vi "svx_DAQ_ConvertState_1000toCurrent.vi"(10 "saved state (version 1.0.0.0)":T1, 11 "current state template":T2 caption="State" {"Timing Control 2" format="%#_6f"; "Channel Info Array"."Max" min=0.0 format="± %^#_4g"; "Channel Info Array"."Channel Type" items=["Voltage (V)"=0, "Charge (C)"=9, "-"=99, "SPL (Pa)"=3, "Force (lbf)"=6, "Force (N)"=1, "Acceleration (g) - IEPE"=2, "Acceleration (g) - Charge"=12, "Acceleration (g) - 4 wire DC Voltage"=22, "Velocity (in/s)"=7, "Velocity (mm/s)"=8, "Prox Probe (mil)"=4, "Prox Probe (mm)"=5]}) -> (3 "Default Control State out":T2 caption="State" {"Timing Control 2" format="%#_6f"; "Channel Info Array"."Max" min=0.0 format="± %^#_4g"; "Channel Info Array"."Channel Type" items=["Voltage (V)"=0, "Charge (C)"=9, "-"=99, "SPL (Pa)"=3, "Force (lbf)"=6, "Force (N)"=1, "Acceleration (g) - IEPE"=2, "Acceleration (g) - Charge"=12, "Acceleration (g) - 4 wire DC Voltage"=22, "Velocity (in/s)"=7, "Velocity (mm/s)"=8, "Prox Probe (mil)"=4, "Prox Probe (mm)"=5]})   [LabVIEW 2017, in "SVX NI-DAQmx AI Configuration XControl.xctl"]
uses:
  <vilib>/addons/Sound and Vibration/svt_DAQmx/Configuration XControl/SVX NI-DAQmx AI Configuration XControl.xctl
  <vilib>/addons/Sound and Vibration/svt_DAQmx/Configuration XControl/SubVIs/svx_DAQ_State.ctl
  <vilib>/addons/Sound and Vibration/svt_DAQmx/Configuration XControl/Controls/svx_DAQ_ChannelInfo.ctl
  <vilib>/addons/Sound and Vibration/svt_DAQmx/Configuration XControl/Controls/svx_DAQ_ChannelType.ctl
  <vilib>/addons/Sound and Vibration/svt_DAQmx/Configuration XControl/Controls/svx_DAQ_Coupling.ctl
  <vilib>/addons/Sound and Vibration/svt_DAQmx/Configuration XControl/Controls/svx_DAQ_Excitation.ctl
  <vilib>/addons/Sound and Vibration/svt_DAQmx/Configuration XControl/Controls/svx_DAQ_TimingType.ctl
  <vilib>/addons/Sound and Vibration/svt_DAQmx/Configuration XControl/Controls/svx_DAQ_ReferenceType.ctl
  <vilib>/addons/Sound and Vibration/svt_DAQmx/Configuration XControl/Controls/svx_DAQ_RotationDirection.ctl
  <vilib>/addons/Sound and Vibration/svt_DAQmx/Configuration XControl/Controls/svx_DAQ_Tach_Slope.ctl
  <vilib>/addons/Sound and Vibration/svt_DAQmx/Configuration XControl/Controls/svx_DAQ_Trigger_Slope.ctl
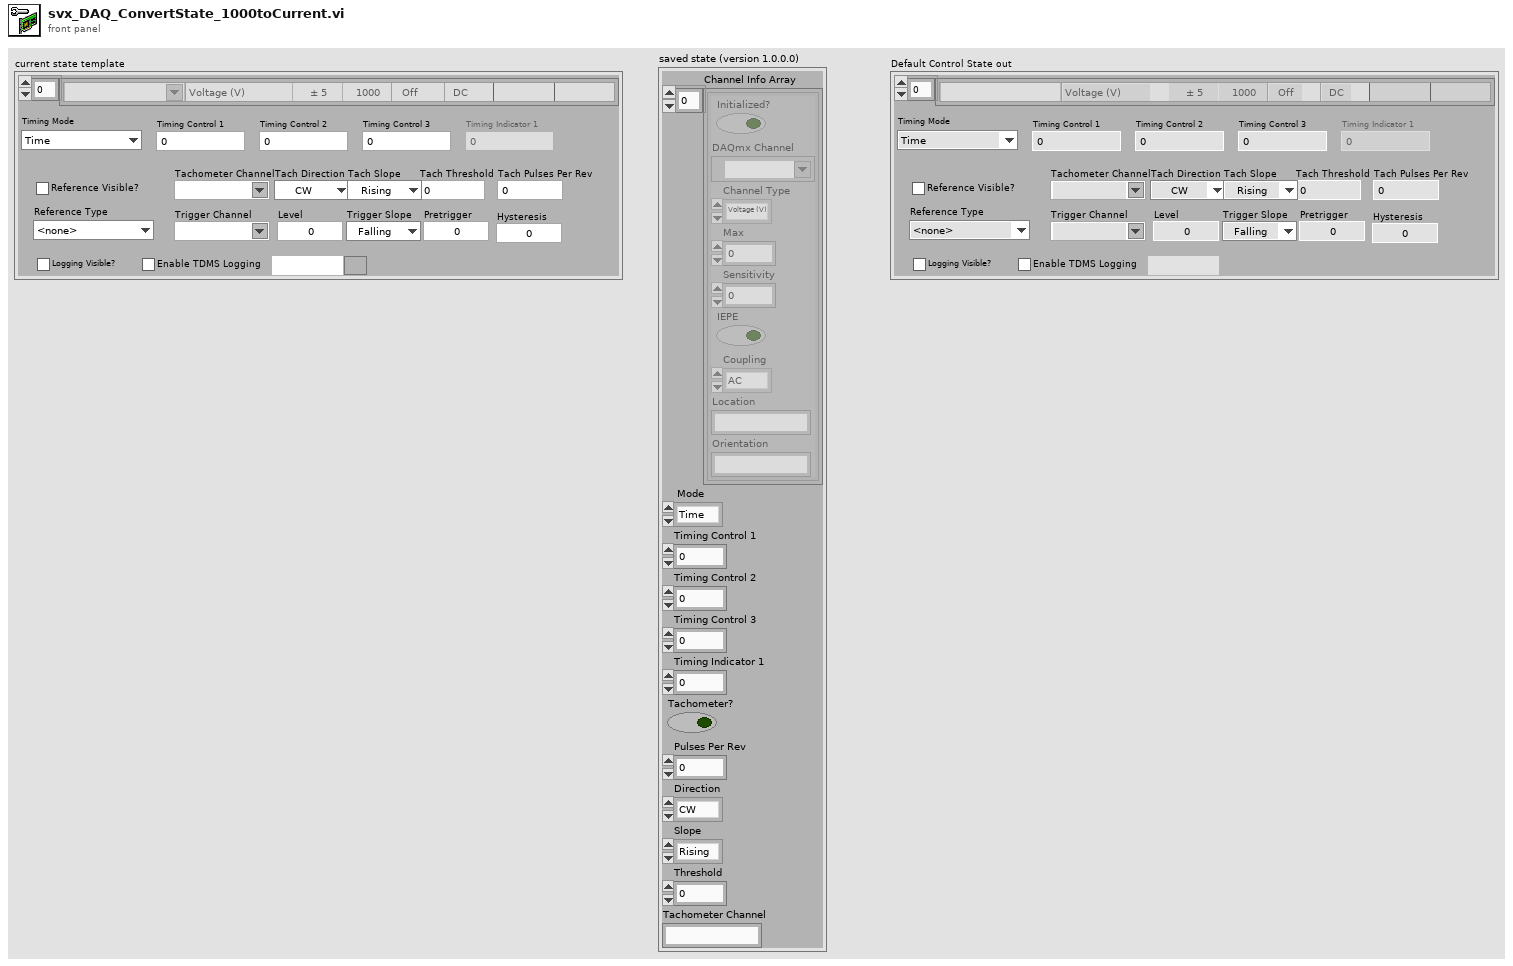
[diagram p1: front panel]
types:
  T1 = cluster{"Channel Info Array":cluster{"Initialized?":bool, "DAQmx Channel":tag, "Channel Type":enum16{"Voltage (V)", "Force (N)", "Acceleration (g)", "SPL (Pa)", "Prox Probe (mil)", "Prox Probe (mm)"}, "Max":dbl, "Sensitivity":dbl, "IEPE":bool, "Coupling":enum16{"AC", "DC"}, "Location":string, "Orientation":string}[], " Mode ":enum16{"Time", "Frequency", "Order"}, "Timing Control 1":dbl, "Timing Control 2":dbl, "Timing Control 3":i32, "Timing Indicator 1":dbl, "Tachometer?":bool, "Pulses Per Rev":i32, "Direction":enum16{"CW", "CCW"}, "Slope":enum16{"Rising", "Falling"}, "Threshold":dbl, "Tachometer Channel":string}
  T2 = typedef "SVX NI-DAQmx AI Configuration XControl.xctl/svx_DAQ_State.ctl" = cluster{"Channel Info Array":T3[], "Timing Mode":T7, "Timing Control 1":dbl, "Timing Control 2":dbl, "Timing Control 3":i32, "Timing Indicator 1":dbl, "Reference Visible?":bool, "Reference Type":T8, "Tachometer Channel":string, "Tach Pulses Per Rev":i32, "Tach Direction":T9, "Tach Slope":T10, "Tach Threshold":dbl, "Trigger Channel":string, "Trigger Level":dbl, "Pretrigger Samples":i32, "Trigger Slope":T11, "Trigger Hysteresis":dbl, "Logging Visible?":bool, "Enable Logging":bool, "Logfile Path":path}
  T3 = typedef "SVX NI-DAQmx AI Configuration XControl.xctl/svx_DAQ_ChannelInfo.ctl" = cluster{"Initialized?":bool, "DAQmx Channel":tag, "Channel Type":T4, "Max":dbl, "Sensitivity":dbl, "Excitation":bool, "Coupling":T5, "Location":string, "Orientation":string, "excitation":T6}
  T4 = typedef "SVX NI-DAQmx AI Configuration XControl.xctl/svx_DAQ_ChannelType.ctl" = u16
  T5 = typedef "SVX NI-DAQmx AI Configuration XControl.xctl/svx_DAQ_Coupling.ctl" = enum16{"AC", "DC"}
  T6 = typedef "svx_DAQ_Excitation.ctl" = enum16{"Off", "Min", "Max"}
  T7 = typedef "SVX NI-DAQmx AI Configuration XControl.xctl/svx_DAQ_TimingType.ctl" = enum16{"Time", "Frequency", "Order"}
  T8 = typedef "SVX NI-DAQmx AI Configuration XControl.xctl/svx_DAQ_ReferenceType.ctl" = enum16{"<none>", "Analog Tachometer", "Analog SW Trigger"}
  T9 = typedef "SVX NI-DAQmx AI Configuration XControl.xctl/svx_DAQ_RotationDirection.ctl" = enum16{"CW", "CCW"}
  T10 = typedef "SVX NI-DAQmx AI Configuration XControl.xctl/svx_DAQ_Tach_Slope.ctl" = enum16{"Rising", "Falling"}
  T11 = typedef "SVX NI-DAQmx AI Configuration XControl.xctl/svx_DAQ_Trigger_Slope.ctl" = enum16{"Falling", "Rising"}
  T12 = cluster{"Initialized?":bool, "DAQmx Channel":tag, "Channel Type":enum16{"Voltage (V)", "Force (N)", "Acceleration (g)", "SPL (Pa)", "Prox Probe (mil)", "Prox Probe (mm)"}, "Max":dbl, "Sensitivity":dbl, "IEPE":bool, "Coupling":enum16{"AC", "DC"}, "Location":string, "Orientation":string}[]
  T13 = enum16{"Voltage (V)", "Force (N)", "Acceleration (g)", "SPL (Pa)", "Prox Probe (mil)", "Prox Probe (mm)"}
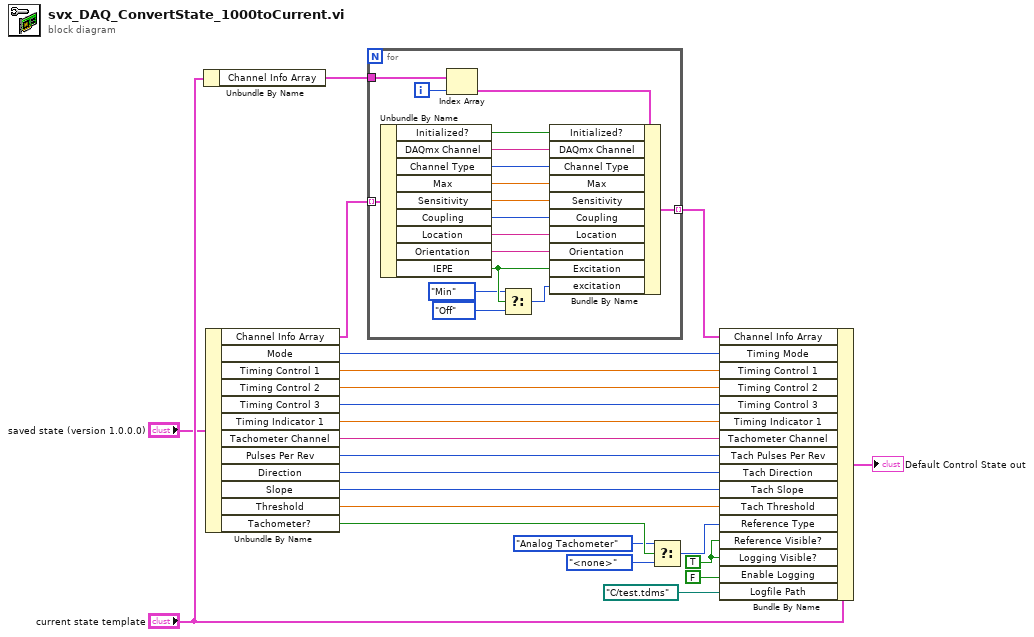
[diagram p0: block diagram]
diagram:
  w15 = TRUE ("Reference Visible?")
  n1 = Unbundle By Name("current state template") -> ("Channel Info Array"=w22:T3[])
  n2 = Unbundle By Name("saved state (version 1.0.0.0)") -> ("Channel Info Array"=w20:T12, "Mode"=w2:enum16{"Time", "Frequency", "Order"}, "Timing Control 1"=w3:dbl, "Timing Control 2"=w4:dbl, "Timing Control 3"=w5:i32, "Timing Indicator 1"=w6:dbl, "Tachometer Channel"=w9:string, "Pulses Per Rev"=w10:i32, "Direction"=w11:enum16{"CW", "CCW"}, "Slope"=w12:enum16{"Rising", "Falling"}, "Threshold"=w13:dbl, "Tachometer?"=w18:bool)
  n3 = for {
    tunnel: w20 -> [w40] mode=indexing
    tunnel: w22 -> [w39]
    tunnel: [w24] -> w23 mode=indexing
    i -> [w38]
    n4 = Unbundle By Name(w40) -> ("Initialized?"=w36:bool, "DAQmx Channel"=w35:tag, "Channel Type"=w34:T13, "Max"=w33:dbl, "Sensitivity"=w32:dbl, "Coupling"=w31:enum16{"AC", "DC"}, "Location"=w30:string, "Orientation"=w29:string, "IEPE"=w28:bool)
    n5 = Index Array(array=w39, index=w38) -> (element=w37:T3)
    n6 = Select(t=svx_DAQ_Excitation."Min" ("excitation"), s=w28, f=svx_DAQ_Excitation."Off" ("excitation")) -> (s? t:f=w25:T6)
    n7 = Bundle By Name(cluster=w37, "Initialized?"=w36, "DAQmx Channel"=w35, "Channel Type"=w34, "Max"=w33, "Sensitivity"=w32, "Coupling"=w31, "Location"=w30, "Orientation"=w29, "Excitation"=w28, "excitation"=w25) -> (w24:T3)
  }
  n8 = Select(t=svx_DAQ_ReferenceType."Analog Tachometer" ("Reference Type"), s=w18, f=svx_DAQ_ReferenceType."<none>" ("Reference Type")) -> (s? t:f=w19:T8)
  n9 = Bundle By Name(cluster="current state template", "Channel Info Array"=w23, "Timing Mode"=w2, "Timing Control 1"=w3, "Timing Control 2"=w4, "Timing Control 3"=w5, "Timing Indicator 1"=w6, "Tachometer Channel"=w9, "Tach Pulses Per Rev"=w10, "Tach Direction"=w11, "Tach Slope"=w12, "Tach Threshold"=w13, "Reference Type"=w19, "Reference Visible?"=w15, "Logging Visible?"=w15, "Enable Logging"=FALSE, "Logfile Path"=path "C:/test.tdms") -> (→"Default Control State out":T2)
